vi "Read Profile Storage Data.vi"(0 "Device ID (0)":i32, 5 "Read Req":T5, 7 "Data Size (0: Auto Size)":u32, 11 "error in (no error)":errorcluster) -> (3 "Profile Info":T1, 4 "Device ID out":i32, 6 "Storage Data":u32[](array[numeric]), 8 "Storage Rsp":T2, 14 "Storage Info":T4, 15 "error out":errorcluster)   [LabVIEW 8.6, in "Keyence LJ-V7000.lvlib"]
doc: "When the storage target setting is profile, this function gets the stored profile data. (Batch setting: off)\n\nIf there is no accumulated data, 0 is output for \"<B>Read Data Cnt</B>\" in <B>Storage Rsp</B>. If the data specified by \"<B>Start Data No</B>\" in <B>Read Req</B> has not been accumulated, one item of the newest data that has been accumulated is returned.\n\n<B>Note</B>:\nFor the details on the data stored in the profile data (storage order and size), see <B>10.3</B> in a manual of measuring instrument drivers."
uses:
  Keyence LJ-V7000.lvlib
  constant/Driver VI No.ctl
  Clusters/Storage Info.ctl
  Clusters/Time.ctl
  Clusters/Read Storage Rsp.ctl
  Private/vi/Low Level/Make DLL Param(Read Storage Rsp).vi
  Private/vi/Low Level/Make VI Param(Read Storage Rsp).vi
  Clusters/Profile Info.ctl
  Clusters/Read Storage Req.ctl
panel:
  # "(c) 2012 KEYENCE CORPORATION.  ALL RIGHTS RESERVED."
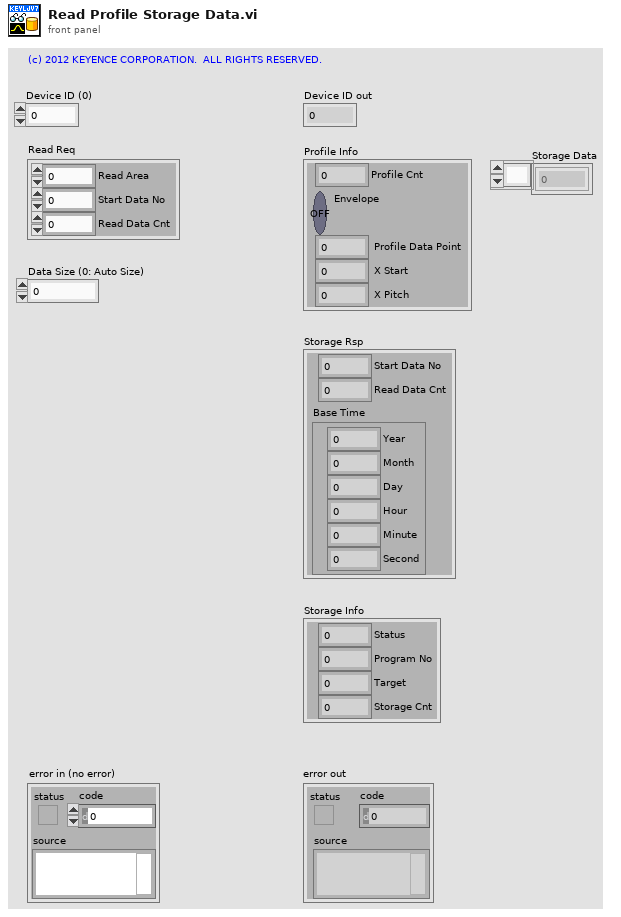
[diagram p1: front panel]
types:
  T1 = typedef "Keyence LJ-V7000.lvlib/Profile Info.ctl" = cluster{"Profile Cnt":u8, "Envelope":bool, " Profile Data Point":u16, " X Start":i32, " X Pitch":i32}
  T2 = typedef "Keyence LJ-V7000.lvlib/Read Storage Rsp.ctl" = cluster{"Start Data No":u32, "Read Data Cnt":u32, "Base Time":T3}
  T3 = typedef "Keyence LJ-V7000.lvlib/Time.ctl" = cluster{"Year":u8, "Month":u8, "Day":u8, "Hour":u8, "Minute":u8, "Second":u8}
  T4 = typedef "Keyence LJ-V7000.lvlib/Storage Info.ctl" = cluster{"Status":u8, "Program No":u8, "Target":u8, "Storage Cnt":u32}
  T5 = typedef "Keyence LJ-V7000.lvlib/Read Storage Req.ctl" = cluster{"Read Area":u32, "Start Data No":u32, "Read Data Cnt":u32}
  T6 = typedef "Keyence LJ-V7000.lvlib/Driver VI No.ctl" = enum16{"Initialize", "Close", "Reboot Controller", "Return to Factory State", "Get System Error", "Clear System Error", "Trigger", "Start Batch Measurements", "Stop Batch Measurements", "Auto Zero", "Timing", "Reset", "Clear Memory", "Set Setting", "Get Setting", "Initialize Setting", "Reflect Setting", "Update Write Settings Area", "Check Status of Saving to Save Area", "Set Time", "Get Time", "Change Program", "Read Active Program Number", "Read Measurement Data", "Read Profiles(for High-Speed Mode)", "Read Batch Profiles(for High-Speed Mode)", "Read Profiles(for Advanced Mode)", "Read Batch Profiles(for Advanced Mode)", "Start Storage", "Stop Storage", "Read Storage Status", "Read Data Storage Data", "Read Profile Storage Data", "Read Batch Profile Storage Data", "Start High-Speed Data Communication", "Stop High-Speed Data Communication", "Read Profiles(for High-Speed Communication)"}
  T7 = cluster{"reserved":u8, "reserved":u8, "reserved":u8, "reserved":u8, "Read Area":u32, "Start Data No":u32, "Read Data Cnt":u32}
  T8 = cluster{"Status":u8, "Program No":u8, "Target":u8, "reserved":u8, "reserved":u8, "reserved":u8, "reserved":u8, "reserved":u8, "Storage Cnt":u32}
  T9 = cluster{"Start Data No":u32, "Read Data Cnt":u32, "pTime":cluster{"Year":u8, "Month":u8, "Day":u8, "Hour":u8, "Minute":u8, "Second":u8, "reserved":u8, "reserved":u8}}
  T10 = cluster{"Profile Cnt":u8, u8, "reserve":u8, "reserve":u8, " Profile Data Point":u16, "reserve":u8, "reserve":u8, " X Start":i32, " XPitch":i32}
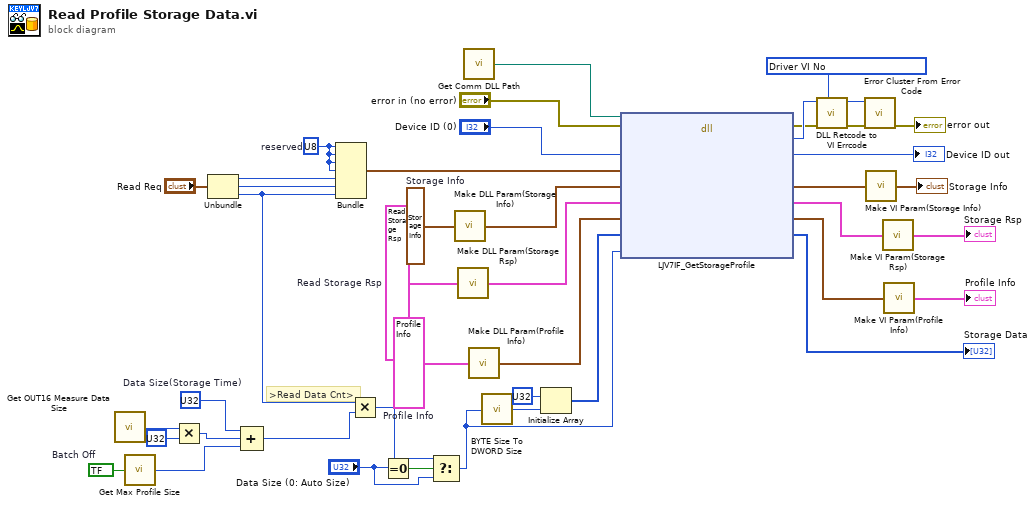
[diagram p0: block diagram]
diagram:
  w19 = bool ?  # Batch Off
  w24 = T1 ?  # Profile Info
  w15 = u32 ?  # Data Size(Storage Time)
  w29 = T2 ?  # Read Storage Rsp
  w33 = T4 ?  # Storage Info
  w35 = u8 ?  # reserved
  # ">Read Data Cnt>"
  n1 = call "Get OUT16 Measure Data Size.vi"() -> ("OUT16 Measure Data Size"=w17:u32)  [unwired: 1 in]
  n2 = call "Get Max Profile Size.vi"("Batch On-Off"=w19) -> ("Profile Size"=w9:u32)  [unwired: 4 in]
  n3 = Multiply(x=w17, y=u32 ?) -> (x*y=w14:u32)
  n4 = Unbundle("Read Req") -> ("Read Area"=w37:u32, "Start Data No"=w36:u32, "Read Data Cnt"=w25:u32)
  n5 = Compound Arithmetic op=ADD(w15, w14, w9) -> (w13:u32)
  n6 = Bundle("reserved"=w35, "reserved"=w35, "reserved"=w35, "reserved"=w35, "Read Area"=w37, "Start Data No"=w36, "Read Data Cnt"=w25) -> (w34:T7)  [unwired: 1 in]
  n7 = Multiply(x=w25, y=w13) -> (x*y=w8:u32)
  n8 = Equal To 0?(x="Data Size (0: Auto Size)") -> (x = 0?=w20:bool)
  n9 = Select(t=w8, s=w20, f="Data Size (0: Auto Size)") -> (s? t:f=w7:u32)
  n10 = call "Make DLL Param(Storage Info).vi"("Storage Info"=w33) -> ("pStorageInfo"=w32:T8)
  n11 = call-poly "Make DLL Param(Storage Rsp).vi"("Read Storage Rsp"=w29) -> ("pRsp"=w28:T9)
  n12 = call "Get Comm DLL Path.vi"() -> ("Comm DLL Path"=w41:path)  [unwired: 1 in]
  n13 = call "Make DLL Param(Profile Info).vi"("Profile Info"=w24) -> ("DLL Parameter"=w23:T10)
  n14 = call "BYTE Size To DWORD Size.vi"("BYTE Size"=w7) -> ("DWORD Size"=w11:u32)
  n15 = Initialize Array(u32 ?, w11) -> (w10:u32[])
  n16 = dll-call lib="C:/Program Files/National Instruments/LabVIEW 2011/instr.lib/Keyence LJ-V7000/LJV7_IF.*" fn="LJV7IF_GetStorageProfile"(path in=w41, error in="error in (no error)", "lDeviceId"="Device ID (0)", "pReq"=w34, "pStorageInfo"=w32, "pRsp"=w28, "pProfileInfo"=w23, "pdwData"=w10, "dwDataSize"=w7) -> (error out=w3:errorcluster, "lRetCode"=w4:i32, "lDeviceId"=→"Device ID out":i32, "pStorageInfo"=w30:T8, "pRsp"=w27:T9, "pProfileInfo"=w21:T10, "pdwData"=→"Storage Data":u32[])  [unwired: 3 in, 1 out]
  n17 = call "DLL Retcode to VI Errcode.vi"("Driver VI No"=T6 ?, "error in (no error)"=w3, "DLL Return Code"=w4) -> ("error out"=w6:errorcluster, "VI Error Code"=w5:i32)  [unwired: 7 in]
  n18 = call <vilib>:"Error Cluster From Error Code.vi"("error in (no error)"=w6, "error code (0)"=w5) -> ("error out"=→"error out":errorcluster)  [unwired: 7 in]
  n19 = call "Make VI Param(Storage Info).vi"("pStorageInfo"=w30) -> ("Storage Info"=→"Storage Info":T4)
  n20 = call-poly "Make VI Param(Storage Rsp).vi"("pRsp"=w27) -> ("Read Storage Rsp"=→"Storage Rsp":T2)
  n21 = call "Make VI Param(Profile Info).vi"("pProfileInfo"=w21) -> ("Profile Info"=→"Profile Info":T1)
